vi "RobotCMD.vi"(3 "Robot Status 2":string="#GetVariable,Message:Pick_Battery_Door") -> (0 "y":dbl format="%#.4f", 1 "x":dbl format="%#.4f")   [LabVIEW 2015]
panel:
  out "2":string
  out "1":string
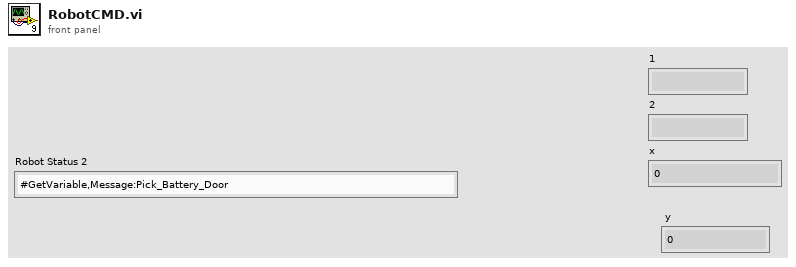
[diagram p1: front panel]
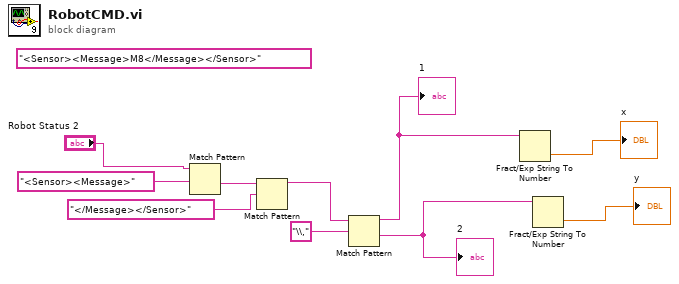
[diagram p0: block diagram]
diagram:
  (unwired) "<Sensor><Message>M8</Message></Sensor>" ("Message")
  n1 = Match Pattern(string="Robot Status 2", regular expression="<Sensor><Message>" ("正则表达式")) -> (after substring=w9:string)  [unwired: 1 in, 3 out]
  n2 = Match Pattern(string=w9, regular expression="</Message></Sensor>" ("正则表达式")) -> (before substring=w5:string)  [unwired: 1 in, 3 out]
  n3 = Match Pattern(string=w5, regular expression="\\," ("正则表达式")) -> (before substring=w4:string, after substring=w1:string)  [unwired: 1 in, 2 out]
  "1" <- w4
  "2" <- w1
  n4 = Fract/Exp String To Number(string=w4) -> (number=→"x":dbl)  [unwired: 3 in, 1 out]
  n5 = Fract/Exp String To Number(string=w1) -> (number=→"y":dbl)  [unwired: 3 in, 1 out]
